vi "Scan action control PPMS2.vi"(0 "Index":i32, 1 "OSC Configuration":T2(array[cluster])=[{"Signal Type"=enum."Sawtooth Wave", "DC"=0.00055, "Amplitude"=0.002, "frequency"=0.25, "Phase"=180.0}, {"Signal Type"=enum."Sine Wave", "DC"=0.0, "Amplitude"=0.0, "frequency"=1.0, "Phase"=0.0}, {"Signal Type"=enum."Sine Wave", "DC"=0.0, "Amplitude"=0.0, "frequency"=1.0, "Phase"=0.0}, {"Signal Type"=enum."Sine Wave", "DC"=0.0, "Amplitude"=0.0, "frequency"=1.0, "Phase"=0.0}] {"frequency" format="%0.2p"; "Amplitude" format="%0.2p"; "DC" format="%.2p"}, 2 "Scan control":u16(ring)=1 items=["OFF", "Vsg1", "Vsg2", "Vsgw", "Vbg", "Field", "Temp", "Position"], 3 "Scan Parameters":T1={"DAQ Channel"=2, "Label"="\nscaledVsg1=", "Scaled low"=-0.060000000000000005, "Scaled high"=0.14, "Start"=0.14, "End"=-0.060000000000000005, "Step"=-0.060000000000000005, "Scale?"=TRUE} {"Step" format="%#_6p"; "End" format="%#_6p"; "Start" format="%#_6p"; "Scaled high" format="%#_6p"; "Scaled low" format="%#_6p"}, 4 "Comments":string) -> (5 "Comments out":string, 6 "OSC Configuration out":T2(array[cluster])=[{"Signal Type"=enum."Sawtooth Wave", "DC"=0.00055, "Amplitude"=0.002, "frequency"=0.25, "Phase"=180.0}, {"Signal Type"=enum."Sine Wave", "DC"=0.0, "Amplitude"=0.0, "frequency"=1.0, "Phase"=0.0}, {"Signal Type"=enum."Sine Wave", "DC"=0.0, "Amplitude"=0.0, "frequency"=1.0, "Phase"=0.0}, {"Signal Type"=enum."Sine Wave", "DC"=0.0, "Amplitude"=0.0, "frequency"=1.0, "Phase"=0.0}] {"frequency" format="%0.2p"; "Amplitude" format="%0.2p"; "DC" format="%.2p"}, 7 "Stop?":bool)   [LabVIEW 2013]
panel:
  in  "Rate (K/min)":dbl=5.0
  in  "Rate (Oe/s)":i32=30
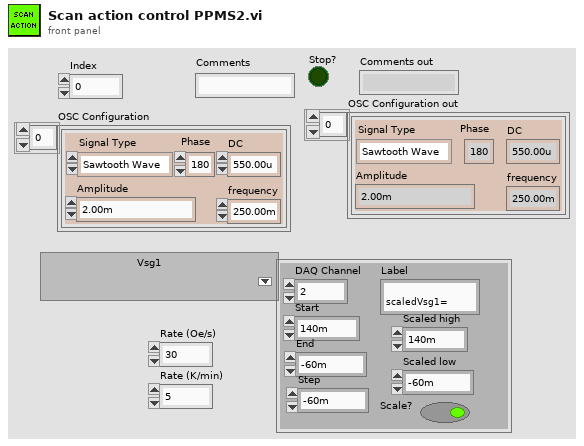
[diagram p1: front panel]
types:
  T1 = cluster{"DAQ Channel":i32, "Label":string, "Scaled low":dbl, "Scaled high":dbl, "Start":dbl, "End":dbl, "Step":dbl, "Scale?":bool}
  T2 = cluster{"Signal Type":enum16{"Sine Wave", "Triangle Wave", "Square Wave", "Sawtooth Wave"}, "DC":dbl, "Amplitude":dbl, "frequency":dbl, "Phase":dbl}[]
  T3 = cluster{"Signal Type":enum16{"Sine Wave", "Triangle Wave", "Square Wave", "Sawtooth Wave"}, "DC":dbl, "Amplitude":dbl, "frequency":dbl, "Phase":dbl}
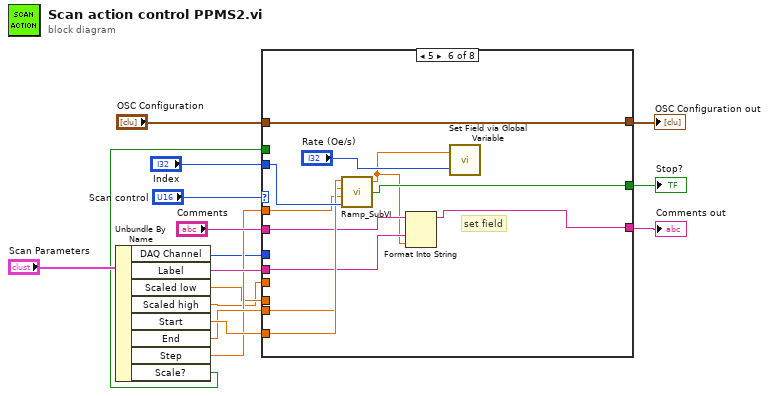
[diagram p0: block diagram]
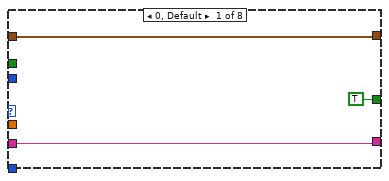
[diagram p2: hidden frame]
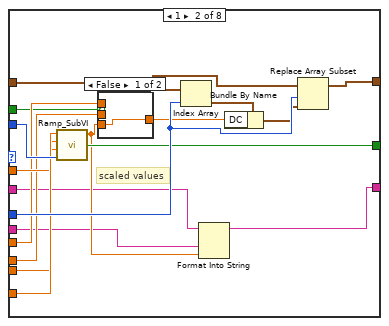
[diagram p3: hidden frame]
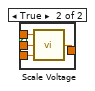
[diagram p4: hidden frame]
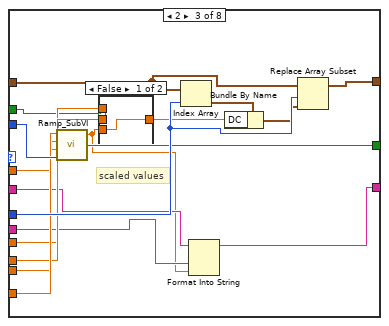
[diagram p5: hidden frame]
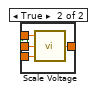
[diagram p6: hidden frame]
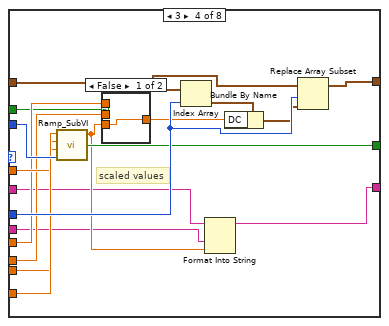
[diagram p7: hidden frame]
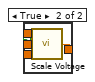
[diagram p8: hidden frame]
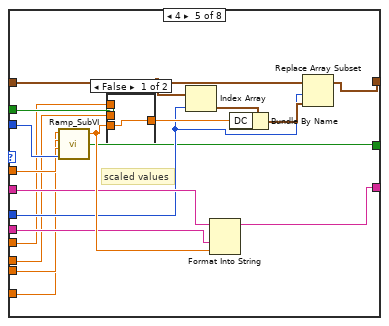
[diagram p9: hidden frame]
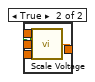
[diagram p10: hidden frame]
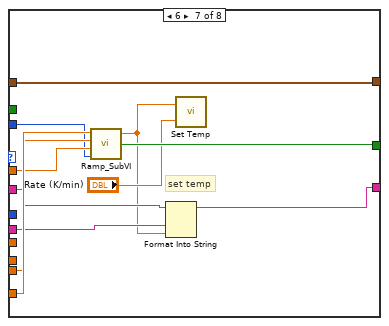
[diagram p11: hidden frame]
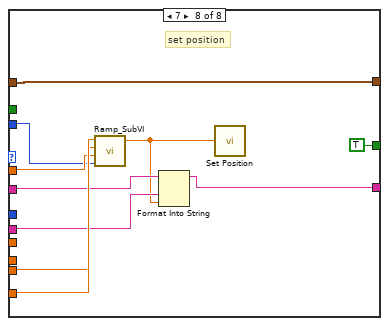
[diagram p12: hidden frame]
diagram:
  n1 = Unbundle By Name("Scan Parameters") -> ("DAQ Channel"=w1:i32, "Label"=w13:string, "Scaled low"=w4:dbl, "Scaled high"=w3:dbl, "Start"=w8:dbl, "End"=w7:dbl, "Step"=w6:dbl, "Scale?"=w2:bool)
  n2 = case shown="5" "Scan control" {
    tunnel: "OSC Configuration" -> [w19 w36 w59 w82 w101 w122 w133 w142]
    tunnel: w1 -> [_ w35 w58 w81 w96 _ _ _]
    tunnel: [w19 w33 w56 w79 w102 w122 w133 w142] -> w12
    tunnel: "Comments" -> [w18 w21 w46 w67 w97 w116 w126 w138]
    tunnel: [w18 w22 w43 w68 w90 w114 w125 w134] -> w11
    tunnel: w13 -> [_ w20 w45 w66 w95 w115 w127 w139]
    tunnel: "Index" -> [_ w32 w55 w78 w99 w121 w129 w136]
    tunnel: w8 -> [_ w31 w54 w77 w91 w120 w132 w141]
    tunnel: w7 -> [_ w30 w53 w76 w92 w119 w131 w140]
    tunnel: w6 -> [_ w29 w52 w75 w98 w118 w130 w137]
    tunnel: [TRUE ("Stop?") w28 w51 w74 w89 w117 w128 TRUE ("Stop?")] -> w5
    tunnel: w4 -> [_ w26 w50 w72 w93 _ _ _]
    tunnel: w3 -> [_ w27 w49 w73 w94 _ _ _]
    tunnel: w2 -> [_ w24 w47 w70 w100 _ _ _]
    frame 0, Default {
    }
    frame 1 {
      # "scaled values"
      n3 = call <userlib>:"Ramp_SubVI.vi"("index"=w32, "step"=w29, "end"=w30, "start"=w31) -> ("Stop?"=w28:bool, "Numeric"=w23:dbl)  [unwired: 1 in]
      n4 = case shown="False" w24 {
        tunnel: w27 -> [_ w42]
        tunnel: w26 -> [_ w41]
        tunnel: w23 -> [w38 w40]
        tunnel: [w38 w39] -> w25
        frame False {
        }
        frame True {
          n5 = call <userlib>:"Scale Voltage.vi"("Scale factor"=w40, "Breakdown Low"=w41, "Breakdown High"=w42) -> ("Real Voltage"=w39:dbl)
        }
      }
      n6 = Index Array(array=w36, index=w35) -> (element=w37:T3)
      n7 = Format Into String(initial string=w21, w20, w23) -> (resulting string=w22:string)  [unwired: 2 in, 1 out]
      n8 = Bundle By Name(cluster=w37, "DC"=w25) -> (w34:T3)
      n9 = Replace Array Subset(array=w36, new element=w34, index=w35) -> (w33:T2)
    }
    frame 2 {
      # "scaled values"
      n10 = call <userlib>:"Ramp_SubVI.vi"("index"=w55, "step"=w52, "end"=w53, "start"=w54) -> ("Stop?"=w51:bool, "Numeric"=w44:dbl)  [unwired: 1 in]
      n11 = case shown="False" w47 {
        tunnel: w50 -> [_ w65]
        tunnel: w49 -> [_ w64]
        tunnel: w44 -> [w61 w63]
        tunnel: [w61 w62] -> w48
        frame False {
        }
        frame True {
          n12 = call <userlib>:"Scale Voltage.vi"("Scale factor"=w63, "Breakdown Low"=w65, "Breakdown High"=w64) -> ("Real Voltage"=w62:dbl)
        }
      }
      n13 = Index Array(array=w59, index=w58) -> (element=w60:T3)
      n14 = Format Into String(initial string=w46, w45, w44) -> (resulting string=w43:string)  [unwired: 2 in, 1 out]
      n15 = Bundle By Name(cluster=w60, "DC"=w48) -> (w57:T3)
      n16 = Replace Array Subset(array=w59, new element=w57, index=w58) -> (w56:T2)
    }
    frame 3 {
      # "scaled values"
      n17 = call <userlib>:"Ramp_SubVI.vi"("index"=w78, "step"=w75, "end"=w76, "start"=w77) -> ("Stop?"=w74:bool, "Numeric"=w69:dbl)  [unwired: 1 in]
      n18 = case shown="False" w70 {
        tunnel: w69 -> [w84 w88]
        tunnel: w73 -> [_ w87]
        tunnel: w72 -> [_ w86]
        tunnel: [w84 w85] -> w71
        frame False {
        }
        frame True {
          n19 = call <userlib>:"Scale Voltage.vi"("Scale factor"=w88, "Breakdown Low"=w86, "Breakdown High"=w87) -> ("Real Voltage"=w85:dbl)
        }
      }
      n20 = Index Array(array=w82, index=w81) -> (element=w83:T3)
      n21 = Format Into String(initial string=w67, w66, w69) -> (resulting string=w68:string)  [unwired: 2 in, 1 out]
      n22 = Bundle By Name(cluster=w83, "DC"=w71) -> (w80:T3)
      n23 = Replace Array Subset(array=w82, new element=w80, index=w81) -> (w79:T2)
    }
    frame 4 {
      # "scaled values"
      n24 = call <userlib>:"Ramp_SubVI.vi"("index"=w99, "step"=w98, "end"=w92, "start"=w91) -> ("Stop?"=w89:bool, "Numeric"=w103:dbl)  [unwired: 1 in]
      n25 = case shown="False" w100 {
        tunnel: w103 -> [w107 w111]
        tunnel: w94 -> [_ w110]
        tunnel: w93 -> [_ w109]
        tunnel: [w107 w108] -> w104
        frame False {
        }
        frame True {
          n26 = call <userlib>:"Scale Voltage.vi"("Scale factor"=w111, "Breakdown Low"=w109, "Breakdown High"=w110) -> ("Real Voltage"=w108:dbl)
        }
      }
      n27 = Index Array(array=w101, index=w96) -> (element=w106:T3)
      n28 = Format Into String(initial string=w97, w95, w103) -> (resulting string=w90:string)  [unwired: 2 in, 1 out]
      n29 = Bundle By Name(cluster=w106, "DC"=w104) -> (w105:T3)
      n30 = Replace Array Subset(array=w101, new element=w105, index=w96) -> (w102:T2)
    }
    frame 5 {
      # "set field"
      n31 = call <userlib>:"Ramp_SubVI.vi"("index"=w121, "step"=w118, "end"=w119, "start"=w120) -> ("Stop?"=w117:bool, "Numeric"=w112:dbl)  [unwired: 1 in]
      n32 = Format Into String(initial string=w116, w115, w112) -> (resulting string=w114:string)  [unwired: 2 in, 1 out]
      n33 = call "Set Field via Global Variable.vi"("Rate"="Rate (Oe/s)", "Field"=w112) -> ()  [unwired: 1 in]
    }
    frame 6 {
      # "set temp"
      n34 = call <userlib>:"Ramp_SubVI.vi"("index"=w129, "step"=w130, "end"=w131, "start"=w132) -> ("Stop?"=w128:bool, "Numeric"=w123:dbl)  [unwired: 1 in]
      n35 = Format Into String(initial string=w126, w127, w123) -> (resulting string=w125:string)  [unwired: 2 in, 1 out]
      n36 = call "Set Temp.vi"("Rate"="Rate (K/min)", "Temperature"=w123) -> ()  [unwired: 1 in]
    }
    frame 7 {
      # "set position"
      n37 = call <userlib>:"Ramp_SubVI.vi"("index"=w136, "step"=w137, "end"=w140, "start"=w141) -> ("Numeric"=w135:dbl)  [unwired: 1 in, 1 out]
      n38 = Format Into String(initial string=w138, w139, w135) -> (resulting string=w134:string)  [unwired: 2 in, 1 out]
      n39 = call "Set Position.vi"("Position"=w135) -> ()  [unwired: 1 in]
    }
  }
  "OSC Configuration out" <- w12
  "Comments out" <- w11
  "Stop?" <- w5
